vi "Configure Park Brake.vi"(8 "error in (no error)":errorcluster, 9 "NIVS.System Definition Root":refnum<k24>, 10 "VI Reference":refnum<vi>, 11 "Park Brake Data in":T1) -> (0 "error out":errorcluster, 3 "Park Brake Data out":T1)   [LabVIEW 2013]
doc: "Use this template to create a dialog box with event handling."
uses:
  NationalInstruments.VeriStand.SystemStorageUI
  NationalInstruments.VeriStand.SystemStorage
  Support/Parking Brake Parameters.ctl
  <vilib>/NI Veristand/UI Controls/Single Node Browser/NI_VS UI Single Node Browser.lvlib
panel:
  in  "Selected Channel -  Ground on Disengage":refnum<k24>(container)
  in  "Lower Pane":u32(colorbox)=1245174
  in  "Upper Pane":u32(colorbox)=1245174
  in  "Control Label":string
  in  "OK":bool
  in  "Cancel":bool
  in  "Selected Channel - Ground on Engage":refnum<k24>(container)
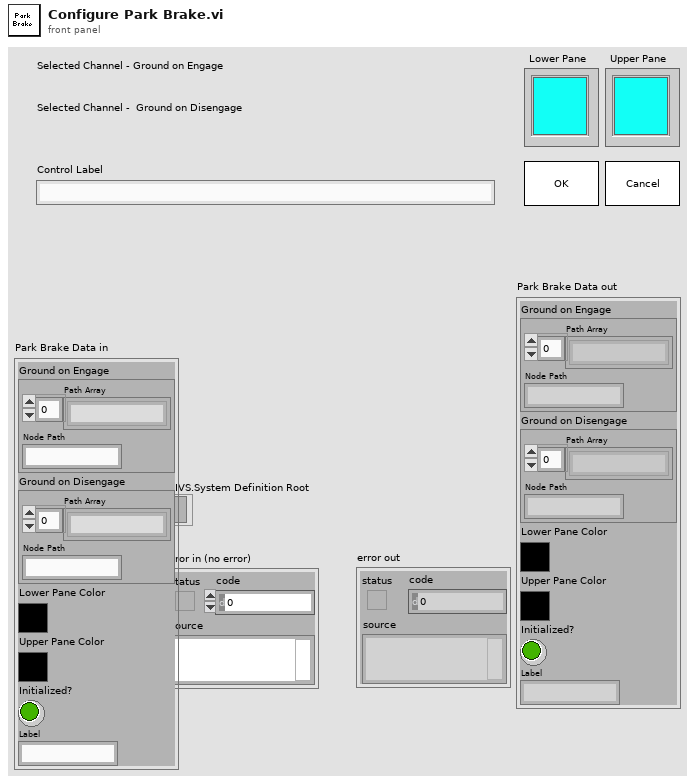
[diagram p1: front panel]
types:
  T1 = typedef "Parking Brake Parameters.ctl" = cluster{"Ground on Engage":cluster{"Path Array":string[], "Node Path":string}, "Ground on Disengage":cluster{"Path Array":string[], "Node Path":string}, "Lower Pane Color":u32, "Upper Pane Color":u32, "Initialized?":bool, "Label":string}
  T2 = typedef "NI_VS UI Single Node Browser.lvlib/Callback Type.ctl" = cluster{"Net Callbacks":refnum<k27>[], "Event":refnum<user-event>}
  T3 = typedef "NI_VS UI Single Node Browser.lvlib/Node Ref.ctl" = refnum<k24>
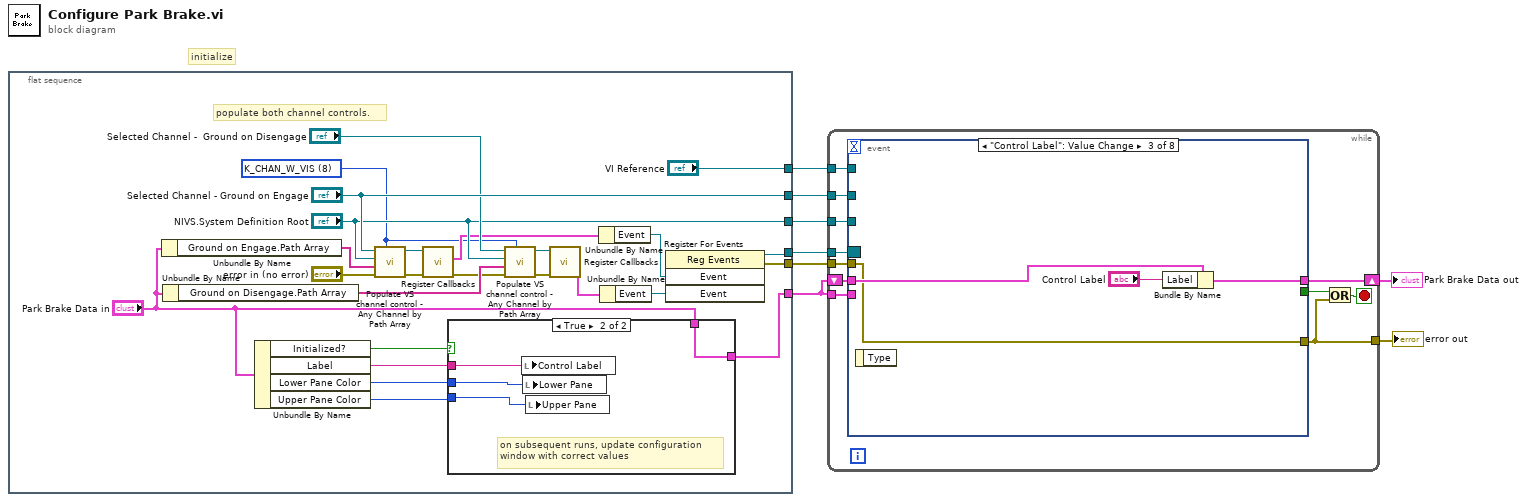
[diagram p0: block diagram]
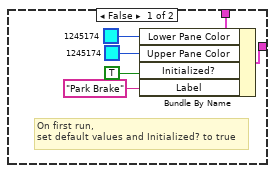
[diagram p2: hidden frame]
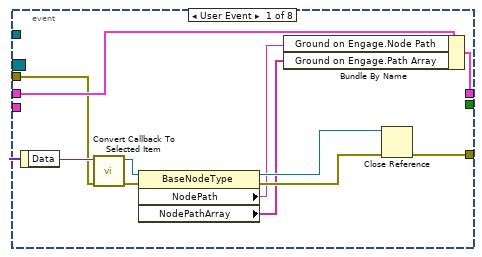
[diagram p3: hidden frame]
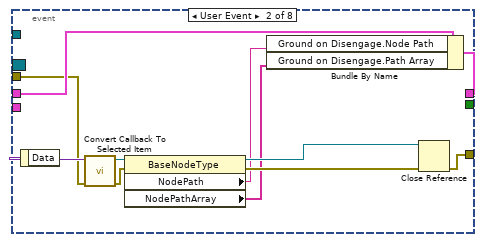
[diagram p4: hidden frame]
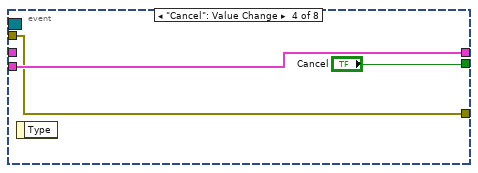
[diagram p5: hidden frame]
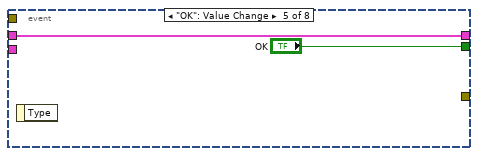
[diagram p6: hidden frame]
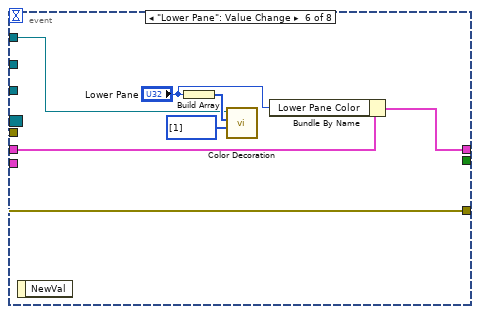
[diagram p7: hidden frame]
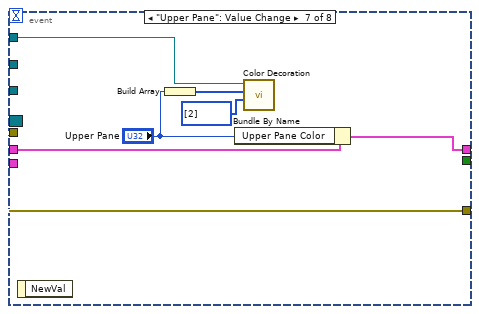
[diagram p8: hidden frame]
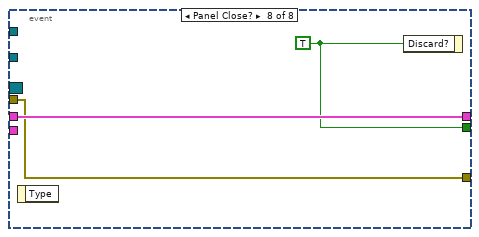
[diagram p9: hidden frame]
diagram:
  # "initialize"
  n1 = flat-sequence {
    tunnel: ["Selected Channel - Ground on Engage"] -> w7
    tunnel: ["NIVS.System Definition Root"] -> w6
    tunnel: [w25] -> w5
    tunnel: [w27] -> w4
    tunnel: ["VI Reference"] -> w3
    tunnel: [w24] -> w2
    frame #0 {
      w9 = u8 8 items=["K_CHAN_R", "K_CHAN_W", "K_CHAN_RW", "K_CHAN_VOLT", "K_CHAN_FAULT", "K_ALL", "K_CUSTOM", "K_CHAN_R_VIS", "K_CHAN_W_VIS", "K_CHAN_RW_VIS", "K_CHAN_VOLT_VIS", "K_CHAN_FAULT_VIS"] ("DisplayFilter")
      # "populate both channel controls."
      n2 = Unbundle By Name("Park Brake Data in") -> ("Ground on Engage.Path Array"=w23:string[])
      n3 = Unbundle By Name("Park Brake Data in") -> ("Ground on Disengage.Path Array"=w22:string[])
      n4 = Unbundle By Name("Park Brake Data in") -> ("Initialized?"=w28:bool, "Label"=w31:string, "Lower Pane Color"=w30:u32, "Upper Pane Color"=w29:u32)
      n5 = call "Populate VS channel control - Any Channel by Path Array.vi"("DisplayFilter"=w9, "error in (no error)"="error in (no error)", "Path Array In"=w23, "NIVS.System Definition Root"="NIVS.System Definition Root", ".NET Refnum in"="Selected Channel - Ground on Engage") -> ("error out"=w14:errorcluster, ".NET Refnum out"=w13:refnum<k24>)  [unwired: 5 in]
      n6 = call <vilib>:"Register Callbacks.vi"("error in (no error)"=w14, "Single Node Browser"=w13) -> ("error out"=w12:errorcluster, "Callbacks"=w11:T2)  [unwired: 7 in, 1 out]
      n7 = case shown="True" w28 {
        tunnel: w31 -> [_ w43]
        tunnel: w30 -> [_ w42]
        tunnel: w29 -> [_ w41]
        tunnel: "Park Brake Data in" -> [w39 w40]
        tunnel: [w38 w40] -> w27
        frame False {
          # "On first run,\nset default values and Initialized? to true"
          n8 = Bundle By Name(cluster=w39, "Lower Pane Color"=u32 1245174, "Upper Pane Color"=u32 1245174, "Initialized?"=TRUE ("New?"), "Label"="Park Brake") -> (w38:T1)
        }
        frame True {
          # "on subsequent runs, update configuration\nwindow with correct values"
          n9 = local write "Control Label"(w43) -> ()
          n10 = local write "Lower Pane"(w42) -> ()
          n11 = local write "Upper Pane"(w41) -> ()
        }
      }
      n12 = call "Populate VS channel control - Any Channel by Path Array.vi"("DisplayFilter"=w9, "error in (no error)"=w12, "Path Array In"=w22, "NIVS.System Definition Root"="NIVS.System Definition Root", ".NET Refnum in"="Selected Channel -  Ground on Disengage") -> ("error out"=w21:errorcluster, ".NET Refnum out"=w20:refnum<k24>)  [unwired: 5 in]
      n13 = call <vilib>:"Register Callbacks.vi"("error in (no error)"=w21, "Single Node Browser"=w20) -> ("Callbacks"=w19:T2)  [unwired: 7 in, 2 out]
      n14 = Unbundle By Name(w11) -> ("Event"=w10:refnum<user-event>)
      n15 = Unbundle By Name(w19) -> ("Event"=w16:refnum<user-event>)
      n16 = register-events(w10, w16) -> (reference out=w24:refnum<event-registration>, error out=w25:errorcluster)  [unwired: 2 in]
    }
  }
  n17 = while {
    tunnel: [w44] -> w8
    shift-right: [w51] -> w1
    shift-left: w4 -> [w53]
    tunnel: w4 -> [w52]
    tunnel: w7 -> [w49]
    tunnel: w6 -> [w48]
    tunnel: w5 -> [w47]
    tunnel: w3 -> [w46]
    tunnel: w2 -> [w45]
    stop <- w50 stop-if-true
    n18 = event shown="[2] \"Control Label\": Value Change" {
      selector: w45 -> [_ _ _ _ _ _ _ _]
      dyn-events: _ -> [_ _ _ _ _ _ _ _]
      timeout: _ -> [_ _ _ _ _ _ _ _]
      tunnel: [_ _ _ "Cancel" "OK" _ _ w101] -> w54
      tunnel: [w57 w68 w77 w81 _ w90 w97 w100] -> w44
      tunnel: w53 -> [w58 w69 w79 _ w84 w91 w98 _]
      tunnel: w52 -> [_ _ _ w82 _ _ _ w102]
      tunnel: [w56 w67 w80 w82 w84 w92 w99 w102] -> w51
      tunnel: w49 -> [_ _ _ _ _ _ _ _]
      tunnel: w48 -> [_ _ _ _ _ _ _ _]
      tunnel: w47 -> [w55 w66 w77 w81 _ w90 w97 w100]
      tunnel: w46 -> [_ _ _ _ _ w87 w93 _]
      event User Event {
        n19 = event-data() -> ("Data"=w59:variant)  [unwired: 1 in]
        n20 = call <vilib>:"Convert Callback To Selected Item.vi"("error in"=w55, "Data"=w59) -> ("error out"=w62:errorcluster, "Selected Item"=w65:T3)  [unwired: 8 in]
        n21 = property class="BaseNodeType"(reference=w65, error in=w62) -> (reference out=w64:T3, error out=w63:errorcluster, "NodePath"=w61:string, "NodePathArray"=w60:string[])
        n22 = Bundle By Name(cluster=w58, "Ground on Engage.Node Path"=w61, "Ground on Engage.Path Array"=w60) -> (w56:T1)
        n23 = Close Reference(reference=w64, error in (no error)=w63) -> (error out=w57:errorcluster)
      }
      event User Event {
        n24 = event-data() -> ("Data"=w70:variant)  [unwired: 1 in]
        n25 = call <vilib>:"Convert Callback To Selected Item.vi"("error in"=w66, "Data"=w70) -> ("error out"=w73:errorcluster, "Selected Item"=w76:T3)  [unwired: 8 in]
        n26 = property class="BaseNodeType"(reference=w76, error in=w73) -> (reference out=w75:T3, error out=w74:errorcluster, "NodePath"=w72:string, "NodePathArray"=w71:string[])
        n27 = Bundle By Name(cluster=w69, "Ground on Disengage.Node Path"=w72, "Ground on Disengage.Path Array"=w71) -> (w67:T1)
        n28 = Close Reference(reference=w75, error in (no error)=w74) -> (error out=w68:errorcluster)
      }
      event "Control Label": Value Change {
        n29 = event-data() -> ()  [unwired: 1 in, 1 out]
        n30 = Bundle By Name(cluster=w79, "Label"="Control Label") -> (w80:T1)
      }
      event "Cancel": Value Change {
        n31 = event-data() -> ()  [unwired: 1 in, 1 out]
      }
      event "OK": Value Change {
        n32 = event-data() -> ()  [unwired: 1 in, 1 out]
      }
      event "Lower Pane": Value Change {
        n33 = event-data() -> ()  [unwired: 1 in, 1 out]
        n34 = Build Array("Lower Pane") -> (w89:u32[])
        n35 = call "Color Decoration.vi"("VI reference"=w87, "Color Array"=w89, "Index Array"=u32[] [1]) -> ()  [unwired: 7 in, 1 out]
        n36 = Bundle By Name(cluster=w91, "Lower Pane Color"="Lower Pane") -> (w92:T1)
      }
      event "Upper Pane": Value Change {
        n37 = event-data() -> ()  [unwired: 1 in, 1 out]
        n38 = Build Array("Upper Pane") -> (w96:u32[])
        n39 = Bundle By Name(cluster=w98, "Upper Pane Color"="Upper Pane") -> (w99:T1)
        n40 = call "Color Decoration.vi"("VI reference"=w93, "Color Array"=w96, "Index Array"=u32[] [2]) -> ()  [unwired: 7 in, 1 out]
      }
      event Panel Close? {
        w101 = TRUE ("Cancel")
        n41 = event-data() -> ()  [unwired: 1 in, 1 out]
        n42 = event-data("Discard?"=w101) -> ()  [unwired: 1 in, 1 out]
      }
    }
    n43 = Or(x=w54, y=w44) -> (x .or. y?=w50:bool)
  }
  "error out" <- w8
  "Park Brake Data out" <- w1
